vi "Billard2023.vi"() -> ()   [LabVIEW 2021]
panel:
  out "standard error C":string
  in  "create Matlab score sheet":bool=TRUE
  in  "Ball diameter":i32=13
  in  "Blue BG":T1={"R max"=62, "R min"=39, "G max"=116, "B max"=255, "B min"=202, "G min"=91}
  in  "White ball":T1={"R max"=255, "R min"=100, "G max"=255, "B max"=250, "B min"=150, "G min"=150}
  in  "Yellow ball":T1={"R max"=255, "R min"=170, "G max"=255, "B max"=175, "B min"=0, "G min"=176}
  in  "Red ball":T1={"R max"=255, "R min"=91, "G max"=80, "B max"=130, "B min"=0, "G min"=0}
  in  "Path":path=path "/Users/mahevelay/Desktop/projet/T4/437.png"
  in  "color loose":u32(colorbox)=16711680
  in  "color win":u32(colorbox)=6618880
  out "standard error ML":string="2023-05-29 17:11:45.354 MATLAB_maci64[56290:2959229] CoreText note: Client requested name \".SFNS-Regular\", it will get Times-Roman rather than the intended font. All system UI font access should be through proper APIs such as CTFontCreateUIFontForLanguage() or +[NSFont systemFontOfSize:].\n2023-05-29 17:11:45.354 MATLAB_maci64[56290:2959229] CoreText note: Set a breakpoint on CTFontLogSystemFontNameRequest to debug.\n2023-05-29 17:11:45.360 MATLAB_maci64[56290:2959229] CoreText note: Client requested name \".SFNS-Bold\", it will get Times-Roman rather than the intended font. All system UI font access should be through proper APIs such as CTFontCreateUIFontForLanguage() or +[NSFont systemFontOfSize:].\n2023-05-29 17:11:45.446 MATLAB_maci64[56290:2959229] CoreText note: Client requested name \".SFNS-Regular\", it will get Times-Roman rather than the intended font. All system UI font access should be through proper APIs such as CTFontCreateUIFontForLanguage() or +[NSFont systemFontOfSize:].\n2023-05-29 17:11:45.447 MATLAB_maci64[56290:2959229] CoreText note: Client requested name \".SFNS-Bold\", it will get Times-Roman rather than the intended font. All system UI font access should be through proper APIs such as CTFontCreateUIFontForLanguage() or +[NSFont systemFontOfSize:].\n"
  out "error out":errorcluster={"status"=TRUE, "code"=-1, "source"="Script error. \n2023-05-29 17:11:45.354 MATLAB_maci64[56290:2959229] CoreText note: Client requested name \".SFNS-Regular\", it will get Times-Roman rather than the intended font. All system UI font access should be through proper APIs such as CTFontCreateUIFontForLanguage() or +[NSFont systemFontOfSize:].\n2023-05-29 17:11:45.354 MATLAB_maci64[56290:2959229] CoreText note: Set a breakpoint on CTFontLogSystemFontNameRequest to debug.\n2023-05-29 17:11:45.360 MATLAB_maci64[56290:2959229] CoreText note: Client requested name \".SFNS-Bold\", it will get Times-Roman rather than the intended font. All system UI font access should be through proper APIs such as CTFontCreateUIFontForLanguage() or +[NSFont systemFontOfSize:].\n2023-05-29 17:11:45.446 MATLAB_maci64[56290:2959229] CoreText note: Client requested name \".SFNS-Regular\", it will get Times-Roman rather than the intended font. All system UI font access should be through proper APIs such as CTFontCreateUIFontForLanguage() or +[NSFont systemFontOfSize:].\n2023-05-29 17:11:45.447 MATLAB_maci64[56290:2959229] CoreText note: Client requested name \".SFNS-Bold\", it will get Times-Roman rather than the intended font. All system UI font access should be through proper APIs such as CTFontCreateUIFontForLanguage() or +[NSFont systemFontOfSize:].\n"}
  in  "dark blue frame":T1={"R max"=24, "R min"=0, "G max"=49, "B max"=119, "B min"=100, "G min"=0}
  out "2D Picture":picture
  in  "line":string=":*"
  # "Billard 2023"
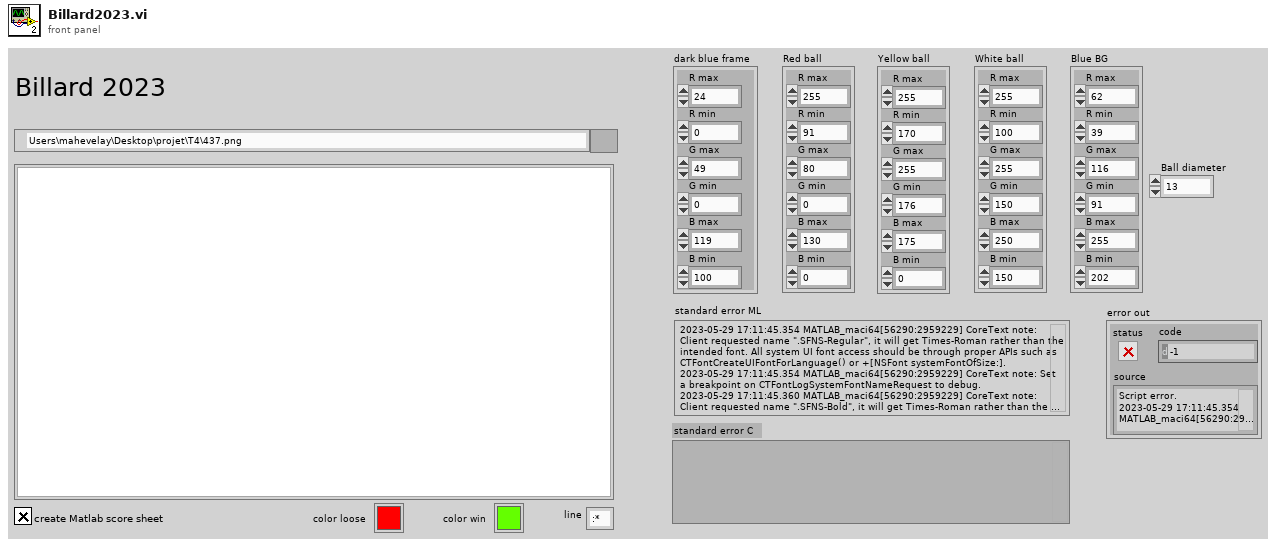
[diagram p1: front panel]
types:
  T1 = cluster{"R max":u8, "R min":u8, "G max":u8, "B max":u8, "B min":u8, "G min":u8}
  T2 = cluster{"left":u32, "top":u32, "right":u32, "bottom":u32}
  T3 = cluster{"Red ball":cluster{"R max":u8, "R min":u8, "G max":u8, "B max":u8, "B min":u8, "G min":u8}, "Yellow ball":cluster{"R max":u8, "R min":u8, "G max":u8, "B max":u8, "B min":u8, "G min":u8}, "White ball":cluster{"R max":u8, "R min":u8, "G max":u8, "B max":u8, "B min":u8, "G min":u8}, "Blue BG":cluster{"R max":u8, "R min":u8, "G max":u8, "B max":u8, "B min":u8, "G min":u8}, "Ball diameter":i32}
  T4 = typedef "imagedata.ctl" = cluster{"image type":i32, "image depth":i32, "image":u8[], "mask":u8[], "colors":u32[], "Rectangle":cluster{"left":i16, "top":i16, "right":i16, "bottom":i16}}
  T5 = enum16{"open", "replace", "create", "open or create", "replace or create", "replace or create with confirmation"}
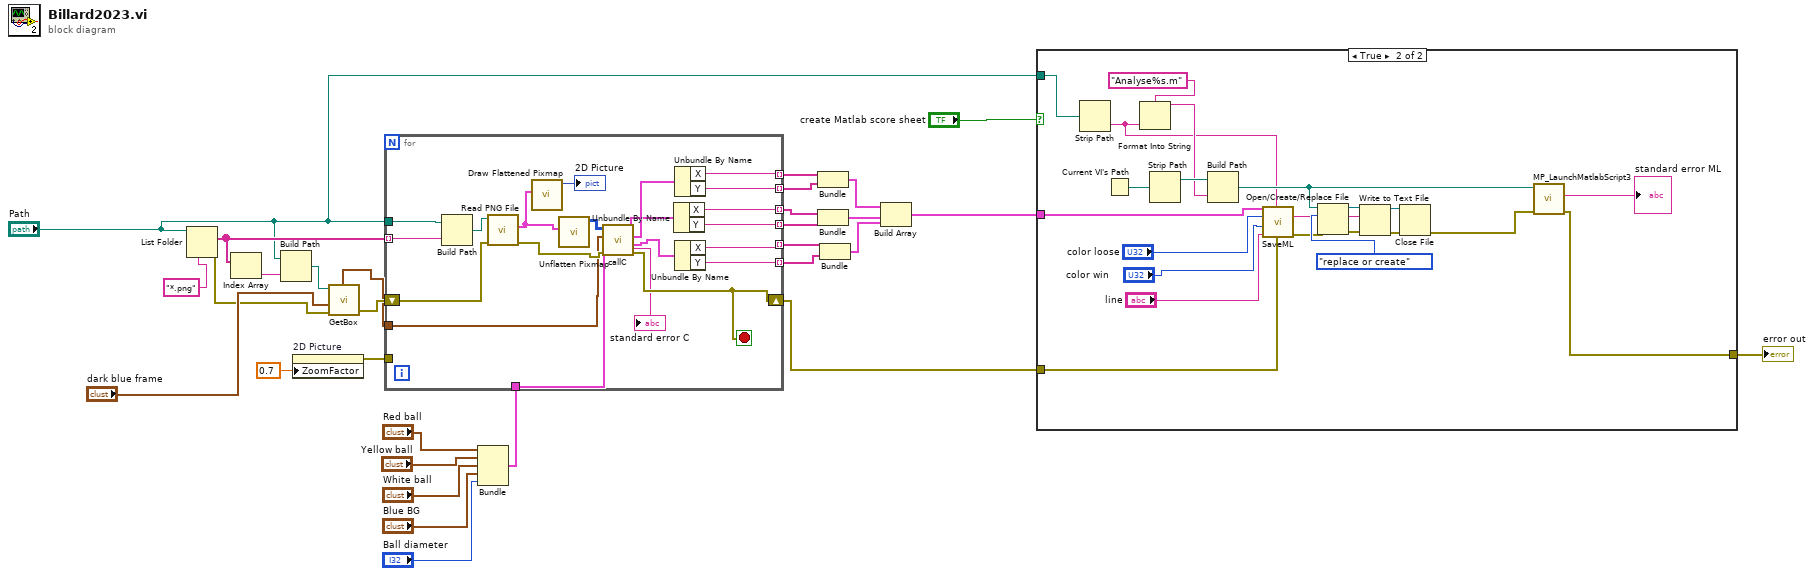
[diagram p0: block diagram]
diagram:
  n1 = List Folder(path="Path", pattern="*.png") -> (filenames=w29:string[], error out=w2:errorcluster)  [unwired: 2 in, 2 out]
  n2 = Index Array(array=w29) -> (element=w28:string)  [unwired: 1 in]
  n3 = Build Path(base path="Path", name or relative path=w28) -> (appended path=w1:path)
  n4 = property on="2D Picture" class="Pict"("ZoomFactor"=0.7) -> (error out=w27:errorcluster)  [unwired: 2 in, 1 out]
  n5 = call "GetBox.vi"("Path"=w1, "dark blue frame"="dark blue frame", "error in"=w2) -> ("billard rect"=w4:T2, "error out"=w5:errorcluster)  [unwired: 3 in]
  n6 = Bundle("Red ball"="Red ball", "Yellow ball"="Yellow ball", "White ball"="White ball", "Blue BG"="Blue BG", "Ball diameter"="Ball diameter") -> (w8:T3)  [unwired: 1 in]
  n7 = for {
    tunnel: w29 -> [w50] mode=indexing
    tunnel: "Path" -> [w51]
    tunnel: w27 -> [_]
    shift-right: [w33] -> w15
    shift-left: w5 -> [w46]
    tunnel: [w42] -> w25 mode=indexing
    tunnel: [w45] -> w24 mode=indexing
    tunnel: [w44] -> w23 mode=indexing
    tunnel: [w43] -> w22 mode=indexing
    tunnel: [w41] -> w21 mode=indexing
    tunnel: [w40] -> w20 mode=indexing
    tunnel: w4 -> [w38]
    tunnel: w8 -> [w32]
    stop <- w33 stop-if-true
    n8 = Build Path(base path=w51, name or relative path=w50) -> (appended path=w49:path)
    n9 = call <vilib>:"Read PNG File.vi"("error in (no error)"=w46, "path to PNG file"=w49) -> ("error out"=w39:errorcluster, "image data"=w47:T4)  [unwired: 7 in, 1 out]
    n10 = call <vilib>:"Draw Flattened Pixmap.vi"("image data"=w47) -> ("new picture"=→"2D Picture":picture)  [unwired: 8 in]
    n11 = call <vilib>:"Unflatten Pixmap.vi"("image data"=w47) -> ("24-bit pixmap"=w37:u32[][])  [unwired: 4 in, 6 out]
    n12 = call "callC.vi"("error in (no error)"=w39, "constant command line"=w32, "billard rect"=w38, "Array"=w37) -> ("error out"=w33:errorcluster, "White"=w34:cluster{"X":string, "Y":string}, "Yellow"=w35:cluster{"X":string, "Y":string}, "Red"=w36:cluster{"X":string, "Y":string}, "standard error"=→"standard error C":string)  [unwired: 2 in, 1 out]
    n13 = Unbundle By Name(w35) -> ("X"=w44:string, "Y"=w43:string)
    n14 = Unbundle By Name(w36) -> ("X"=w42:string, "Y"=w45:string)
    n15 = Unbundle By Name(w34) -> ("X"=w41:string, "Y"=w40:string)
  }
  n16 = Bundle(w25, w24) -> (w19:cluster{string[], string[]})  [unwired: 1 in]
  n17 = Bundle(w23, w22) -> (w18:cluster{string[], string[]})  [unwired: 1 in]
  n18 = Bundle(w21, w20) -> (w17:cluster{string[], string[]})  [unwired: 1 in]
  n19 = Build Array(w19, w18, w17) -> (w16:cluster{string[], string[]}[])
  n20 = case shown="True" "create Matlab score sheet" {
    tunnel: w16 -> [_ w59]
    tunnel: w15 -> [w52 w53]
    tunnel: "Path" -> [_ w74]
    tunnel: [w52 w62] -> w14
    frame False {
    }
    frame True {
      n21 = Strip Path(path=w74) -> (name=w58:string)  [unwired: 1 out]
      n22 = Current VI's Path() -> (path=w73:path)
      n23 = Format Into String(format string="Analyse%s.m", w58) -> (resulting string=w71:string)  [unwired: 2 in, 1 out]
      n24 = Strip Path(path=w73) -> (stripped path=w72:path)  [unwired: 1 out]
      n25 = Build Path(base path=w72, name or relative path=w71) -> (appended path=w64:path)
      n26 = call "SaveML.vi"("error in"=w53, "Nom de la sequence"=w58, "line"="line", "color win"="color win", "color loose"="color loose", "Pos"=w59) -> ("error out"=w60:errorcluster, "script ML"=w57:string)  [unwired: 4 in]
      n27 = Open/Create/Replace File(file path (use dialog)=w64, error in=w60, operation (0:open)=T5."replace or create") -> (refnum out=w68:refnum<file>, error out=w69:errorcluster)  [unwired: 3 in, 1 out]
      n28 = Write to Text File(file (use dialog)=w68, text=w57, error in=w69) -> (refnum out=w66:refnum<file>, error out=w67:errorcluster)  [unwired: 1 in, 1 out]
      n29 = Close File(refnum=w66, error in=w67) -> (error out=w63:errorcluster)  [unwired: 1 out]
      n30 = call "MP_LaunchMatlabScript3.vi"("error in (no error)"=w63, "matlab script with path"=w64) -> ("error out"=w62:errorcluster, "standard error"=→"standard error ML":string)  [unwired: 5 in, 3 out]
    }
  }
  "error out" <- w14
